vi "Handle Errors.vi"(8 "error in (no error)":errorcluster) -> (0 "error out":errorcluster)   [LabVIEW 2020, in "Error Handler.lvclass"]
uses:
  Error Handler.lvclass
  Error Handler.lvclass/Error Handler.ctl
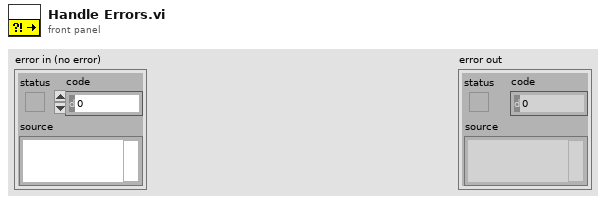
[diagram p1: front panel]
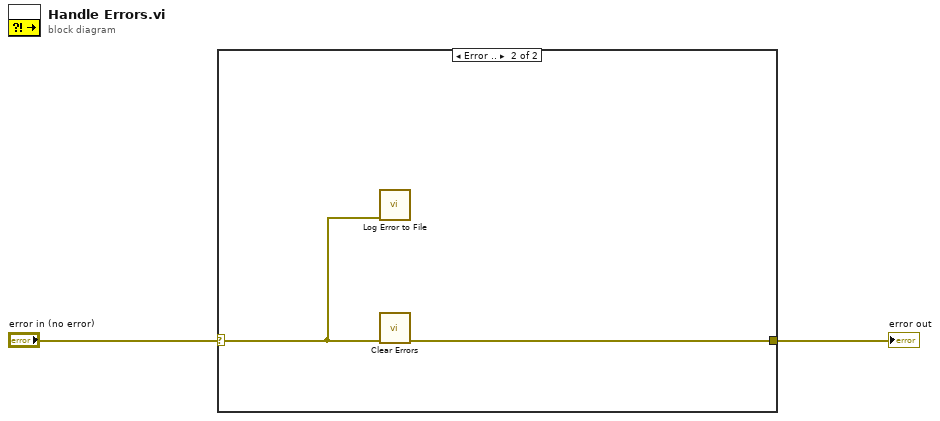
[diagram p0: block diagram]
diagram:
  n1 = case shown="Error .." "error in (no error)" {
    selector: "error in (no error)" -> [w3 w4]
    tunnel: [w3 w5] -> w1
    frame No Error {
    }
    frame Error {
      n2 = call "Log Error to File.vi"("error in (no error)"=w4) -> ()  [unwired: 11 in]
      n3 = call <vilib>:"Clear Errors.vi"("error in (no error)"=w4) -> ("error out"=w5:errorcluster)  [unwired: 5 in, 1 out]
    }
  }
  "error out" <- w1
